vi "_04_import a S-VI in while loop and shown the example in wave form.vi"() -> ()   [LabVIEW 2020]
panel:
  out "Waveform Chart 4":dbl(graph)
  out "Waveform Chart 3":dbl(graph)
  out "Waveform Chart 2":dbl(graph)
  out "Waveform Chart":dbl(graph)
  # "Fluctuate"
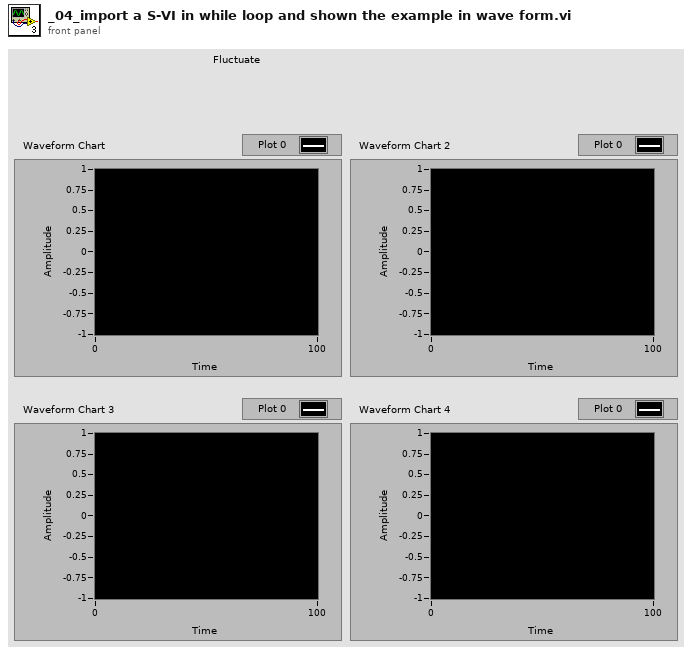
[diagram p1: front panel]
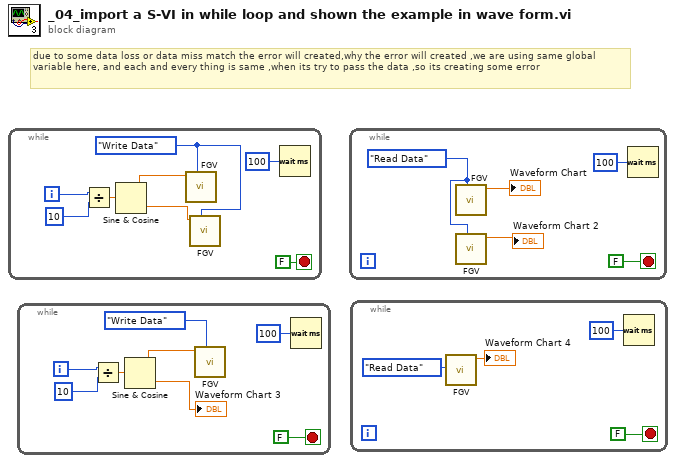
[diagram p0: block diagram]
diagram:
  # "due to some data loss or data miss match the error will created,why the error will created ,we are using same global \nvariable here, and each and every thing is same ,when its try to pass the data ,so its creating some error"
  n1 = while {
    i -> [w7]
    stop <- FALSE stop-if-true
    w5 = enum16{"Read Data", "Write Data"}."Write Data" ("Enum")
    n2 = Divide(x=w7, y=10) -> (x/y=w8:dbl)
    n3 = Sine & Cosine(0:w8) -> (1:w4:dbl, 2:w3:dbl)
    n4 = call "FGV.vi"("Enum"=w5, "i/p"=w4) -> ()  [unwired: 8 in, 2 out]
    n5 = call "FGV.vi"("Enum"=w5, "i/p"=w3) -> ()  [unwired: 8 in, 2 out]
    n6 = Wait (ms)(milliseconds to wait=u32 100 ("millisecond timer value")) -> ()  [unwired: 1 out]
  }
  n7 = while {
    i -> [w15]
    stop <- FALSE stop-if-true
    n8 = Divide(x=w15, y=10) -> (x/y=w16:dbl)
    n9 = Sine & Cosine(0:w16) -> (1:w11:dbl, 2:→"Waveform Chart 3":dbl)
    n10 = call "FGV.vi"("Enum"=enum16{"Read Data", "Write Data"}."Write Data", "i/p"=w11) -> ()  [unwired: 8 in, 2 out]
    n11 = Wait (ms)(milliseconds to wait=u32 100 ("millisecond timer value")) -> ()  [unwired: 1 out]
  }
  n12 = while {
    stop <- FALSE stop-if-true
    w17 = enum16{"Read Data", "Write Data"}."Read Data" ("Enum")
    n13 = call "FGV.vi"("Enum"=w17) -> ("o/p"=→"Waveform Chart":dbl)  [unwired: 9 in, 1 out]
    n14 = call "FGV.vi"("Enum"=w17) -> ("o/p"=→"Waveform Chart 2":dbl)  [unwired: 9 in, 1 out]
    n15 = Wait (ms)(milliseconds to wait=u32 100 ("millisecond timer value")) -> ()  [unwired: 1 out]
  }
  n16 = while {
    stop <- FALSE stop-if-true
    n17 = call "FGV.vi"("Enum"=enum16{"Read Data", "Write Data"}."Read Data") -> ("o/p"=→"Waveform Chart 4":dbl)  [unwired: 9 in, 1 out]
    n18 = Wait (ms)(milliseconds to wait=u32 100 ("millisecond timer value")) -> ()  [unwired: 1 out]
  }
